vi "WireCaseStructure.vi"(6 "Error terminals":T1, 8 "error in (no error)":errorcluster, 10 "New case structure ref":refnum<vi>, 11 "VI ref in":refnum<vi>) -> (0 "error out":errorcluster, 3 "VI ref out (dup)":refnum<vi>)   [LabVIEW 2017, in "ErrorStructureDrawer.lvlib"]
doc: "Moves the case structure's outer terminal to the correct vertical position for wire alignment with the error control, and draws a wire between them, and between the terminal and the error indicator (through the \"Error\" case).\n\nAlso cleans wires outside the case structure."
uses:
  ErrorStructureDrawer.lvlib
  Controls/ErrorTerminals.ctl
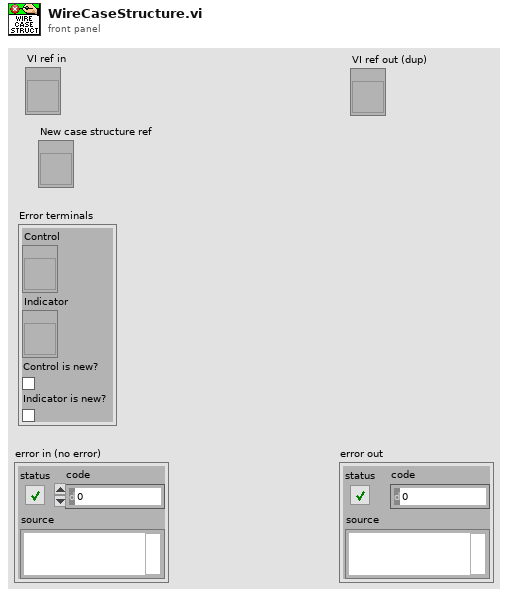
[diagram p1: front panel]
types:
  T1 = typedef "ErrorStructureDrawer.lvlib/ErrorTerminals.ctl" = cluster{"Control":refnum<vi>, "Indicator":refnum<vi>, "Control is new?":bool, "Indicator is new?":bool}
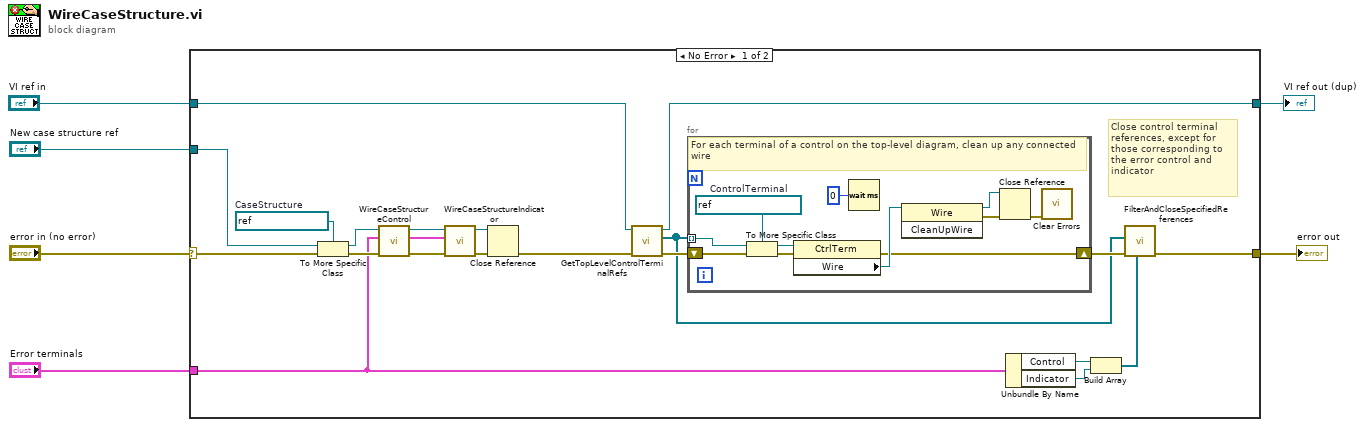
[diagram p0: block diagram]
diagram:
  n1 = case shown="No Error" "error in (no error)" {
    selector: "error in (no error)" -> [w18 w40]
    tunnel: [w16 w40] -> w6
    tunnel: "New case structure ref" -> [w24 _]
    tunnel: "Error terminals" -> [w10 _]
    tunnel: "VI ref in" -> [w13 w39]
    tunnel: [w12 w39] -> w1
    frame No Error {
      w25 = refnum<vi> refnum  # CaseStructure
      # "Close control terminal references, except for those corresponding to the error control and indicator"
      n2 = To More Specific Class(target class=w25, reference=w24, error in=w18) -> (specific class reference=w23:refnum<vi>, error out=w22:errorcluster)
      n3 = call "WireCaseStructureControl.vi"("error in (no error)"=w22, "Error terminals"=w10, "Case structure"=w23) -> ("error out"=w26:errorcluster, "Error terminals (dup)"=w21:T1, "CaseStructure (dup)"=w27:refnum<vi>)  [unwired: 6 in]
      n4 = call "WireCaseStructureIndicator.vi"("error in (no error)"=w26, "Error terminals"=w21, "CaseStructure in"=w27) -> ("error out"=w20:errorcluster, "CaseStructure (dup)"=w19:refnum<vi>)  [unwired: 6 in, 1 out]
      n5 = Close Reference(reference=w19, error in (no error)=w20) -> (error out=w14:errorcluster)
      n6 = call "GetTopLevelControlTerminalRefs.vi"("error in (no error)"=w14, "VI ref in"=w13) -> ("error out"=w15:errorcluster, "Control terminals on top-level"=w11:refnum<vi>[], "VI ref out (dup)"=w12:refnum<vi>)  [unwired: 7 in]
      n7 = for {
        tunnel: w11 -> [w37] mode=indexing
        shift-right: [w30] -> w17
        shift-left: w15 -> [w38]
        w36 = refnum<vi> refnum  # ControlTerminal
        # "For each terminal of a control on the top-level diagram, clean up any connected wire"
        n8 = To More Specific Class(target class=w36, reference=w37, error in=w38) -> (specific class reference=w34:refnum<vi>, error out=w35:errorcluster)
        n9 = property class="CtrlTerm"(reference=w34, error in=w35) -> (error out=w30:errorcluster, "Wire"=w33:refnum<vi>)  [unwired: 1 out]
        n10 = Wait (ms)(milliseconds to wait=u32 0) -> ()  [unwired: 1 out]
        n11 = invoke class="Wire" method="CleanUpWire"(reference=w33) -> (reference out=w31:refnum<vi>, error out=w32:errorcluster)  [unwired: 2 in, 1 out]
        n12 = Close Reference(reference=w31, error in (no error)=w32) -> (error out=w29:errorcluster)
        n13 = call <vilib>:"Clear Errors.vi"("error in (no error)"=w29) -> ()  [unwired: 5 in, 2 out]
      }
      n14 = Unbundle By Name(w10) -> ("Control"=w9:refnum<vi>, "Indicator"=w7:refnum<vi>)
      n15 = Build Array(w9, w7) -> (w8:refnum<vi>[])
      n16 = call "FilterAndCloseSpecifiedReferences.vi"("Control references to filter"=w8, "error in (no error)"=w17, "Control references to close"=w11) -> ("error out"=w16:errorcluster)  [unwired: 8 in]
    }
    frame Error {
    }
  }
  "error out" <- w6
  "VI ref out (dup)" <- w1
